vi "calculos_acel_desl_velo.vi"(9 "Numeric Control":dbl, 10 "TimeStamp":dbl, 11 "Joints":dbl[](array[numeric])) -> (1 "Aceleração":dbl[](array[numeric]), 2 "Velocidade":dbl[](array[numeric]), 3 "Deslocamento":dbl[](array[numeric]))   [LabVIEW 2016]
uses:
  Software_TCC/historico_dados.vi
panel:
  out "último Valor":dbl[](array[numeric])
  out "Aceleração":dbl[](array[numeric])
  out "Velocidade":dbl[](array[numeric])
  out "Deslocamento":dbl[](array[numeric])
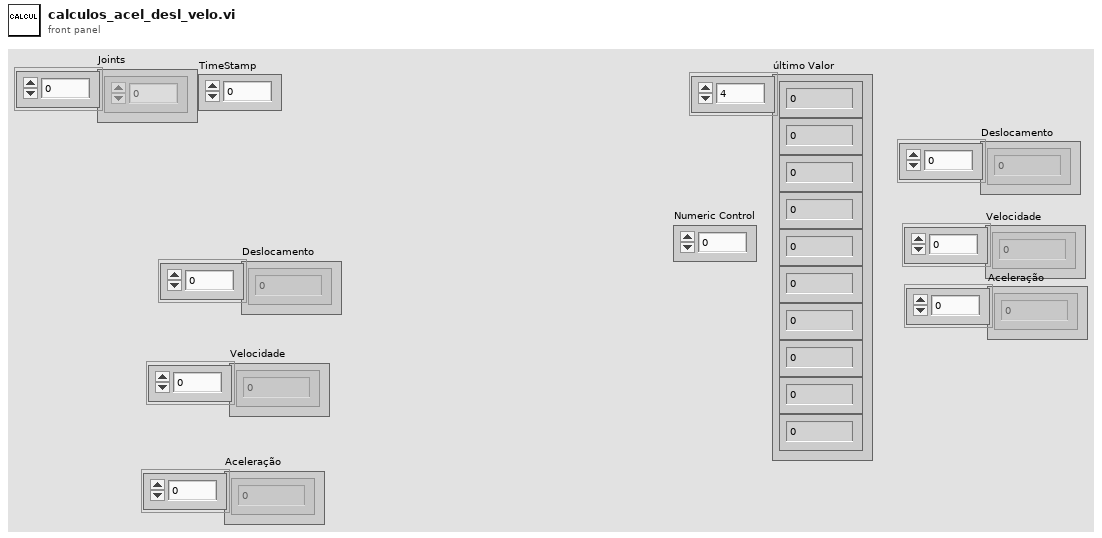
[diagram p1: front panel]
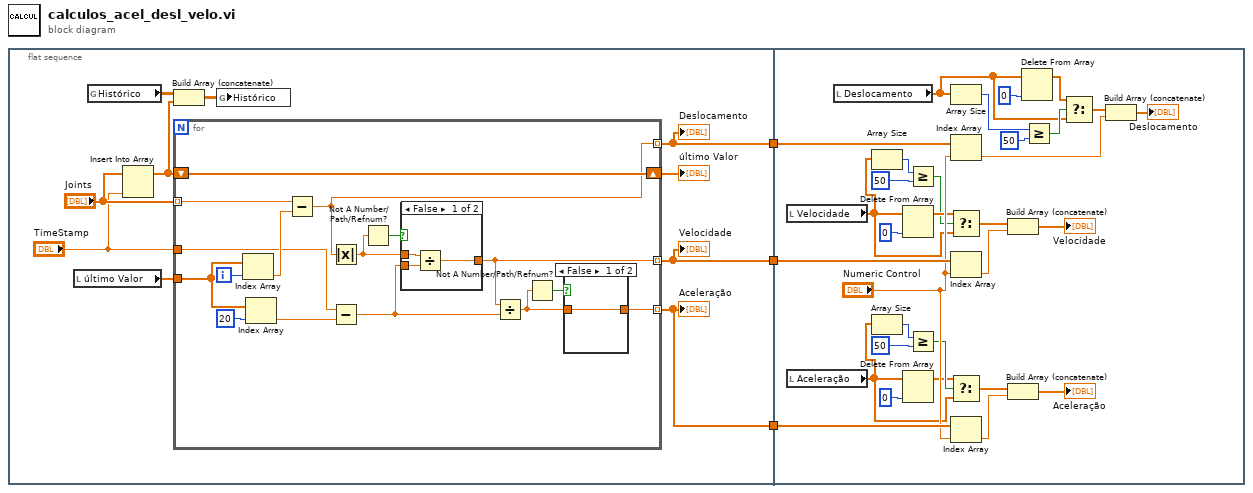
[diagram p0: block diagram]
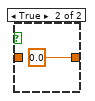
[diagram p2: hidden frame]
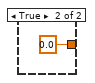
[diagram p3: hidden frame]
diagram:
  n1 = flat-sequence {
    tunnel: [w6] -> w3
    tunnel: [w5] -> w2
    tunnel: [w4] -> w1
    tunnel: w3 -> [w66]
    tunnel: w2 -> [w65]
    tunnel: w1 -> [w64]
    frame #0 {
      n2 = local read "último Valor"() -> (w10:dbl[])
      n3 = global read "historico_dados.vi" "Histórico"() -> (w13:dbl[][])
      n4 = Insert Into Array(array="Joints", new element="TimeStamp") -> (w8:dbl[])  [unwired: 1 in]
      n5 = Build Array (concatenate)(w13, w8) -> (w12:dbl[][])
      n6 = for {
        tunnel: "Joints" -> [w29] mode=indexing
        tunnel: w10 -> [w26]
        tunnel: [w20] -> w6 mode=indexing
        tunnel: "TimeStamp" -> [w24]
        tunnel: [w17] -> w5 mode=indexing
        tunnel: [w22] -> w4 mode=indexing
        shift-right: [w21] -> w7
        shift-left: w8 -> [w21]
        i -> [w28]
        n7 = Index Array(array=w26, index=w28) -> (element=w27:dbl)
        n8 = Index Array(array=w26, index=20) -> (element=w23:dbl)
        n9 = Subtract(x=w29, y=w27) -> (x-y=w20:dbl)
        n10 = Absolute Value(x=w20) -> (abs(x)=w19:dbl)
        n11 = Subtract(x=w24, y=w23) -> (x-y=w16:dbl)
        n12 = Not A Number/Path/Refnum?(number/path/refnum=w19) -> (NaN/Path/Refnum?=w18:bool)
        n13 = case shown="False" w18 {
          tunnel: [w34 0.0] -> w17
          tunnel: w16 -> [w33 _]
          tunnel: w19 -> [w32 _]
          frame False {
            n14 = Divide(x=w32, y=w33) -> (x/y=w34:dbl)
          }
          frame True {
          }
        }
        n15 = Divide(x=w17, y=w16) -> (x/y=w14:dbl)
        n16 = Not A Number/Path/Refnum?(number/path/refnum=w14) -> (NaN/Path/Refnum?=w15:bool)
        n17 = case shown="False" w15 {
          tunnel: [w30 0.0] -> w22
          tunnel: w14 -> [w30 _]
          frame False {
          }
          frame True {
          }
        }
      }
      "Deslocamento" <- w6
      "Velocidade" <- w5
      "Aceleração" <- w4
      "último Valor" <- w7
      n18 = global write "historico_dados.vi" "Histórico"(w12) -> ()
    }
    frame #1 {
      n19 = local read "Velocidade"() -> (w36:dbl[])
      n20 = local read "Aceleração"() -> (w37:dbl[])
      n21 = local read "Deslocamento"() -> (w38:dbl[])
      n22 = Array Size(array=w36) -> (size(s)=w46:i32)
      n23 = Array Size(array=w37) -> (size(s)=w45:i32)
      n24 = Delete From Array(array=w36, index=0) -> (array with subset deleted=w49:dbl[])  [unwired: 1 in, 1 out]
      n25 = Delete From Array(array=w37, index=0) -> (array with subset deleted=w42:dbl[])  [unwired: 1 in, 1 out]
      n26 = Greater Or Equal?(x=w46, y=50) -> (x >= y?=w48:bool)
      n27 = Greater Or Equal?(x=w45, y=50) -> (x >= y?=w43:bool)
      n28 = Array Size(array=w38) -> (size(s)=w56:i32)
      n29 = Index Array(array=w66, index="Numeric Control") -> (element=w62:dbl)
      n30 = Select(t=w49, s=w48, f=w36) -> (s? t:f=w40:dbl[])
      n31 = Index Array(array=w65, index="Numeric Control") -> (element=w61:dbl)
      n32 = Select(t=w42, s=w43, f=w37) -> (s? t:f=w39:dbl[])
      n33 = Index Array(array=w64, index="Numeric Control") -> (element=w60:dbl)
      n34 = Build Array (concatenate)(w40, w61) -> (→"Velocidade":dbl[])
      n35 = Build Array (concatenate)(w39, w60) -> (→"Aceleração":dbl[])
      n36 = Delete From Array(array=w38, index=0) -> (array with subset deleted=w53:dbl[])  [unwired: 1 in, 1 out]
      n37 = Greater Or Equal?(x=w56, y=50) -> (x >= y?=w54:bool)
      n38 = Select(t=w53, s=w54, f=w38) -> (s? t:f=w51:dbl[])
      n39 = Build Array (concatenate)(w51, w62) -> (→"Deslocamento":dbl[])
    }
  }
